vi "Read User Devices.vi"(8 "error in (no error)":errorcluster, 11 "Platforms":refnum<class "PlatformManager.lvclass">) -> (0 "error out":errorcluster, 3 "User Devices":refnum<class "Device.lvclass">[](array[class]))   [LabVIEW 2020, in "PicoG-App.lvlib" / "picoG.lvclass"]
uses:
  picoG.lvclass
  Device/Device.lvclass
  Builds/picoG/ppl/PicoG-Core.lvlibp/PicoG-Processor/PicoG-Core/PlatformManager/PlatformManager.lvclass
  <vilib>/Utility/config.llb/Read Key (I32).vi
  PicoG-App.lvlib
  <vilib>/Utility/config.llb/NI_LVConfig.lvlib
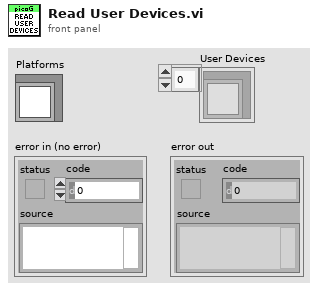
[diagram p1: front panel]
types:
  T1 = typedef "PicoG-App.lvlib/Paths.ctl" = cluster{"User picoG":path, "System picoG":path, "User Config":path, "System Config":path}
  T2 = typedef "NI_LVConfig.lvlib/Config Data RefNum.ctl" = refnum<k1>
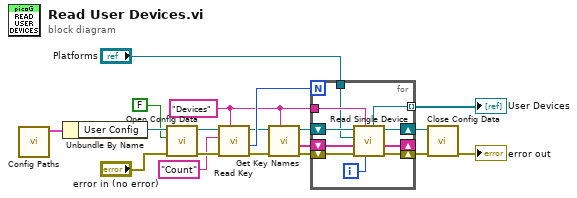
[diagram p0: block diagram]
diagram:
  w2 = "Devices" ("key")
  n1 = call "Config Paths.vi"() -> ("Paths"=w19:T1)  [unwired: 8 in, 3 out]
  n2 = Unbundle By Name(w19) -> ("User Config"=w18:path)
  n3 = call <vilib>:"Open Config Data.vi"("error in (no error)"="error in (no error)", "create file if necessary (T)"=FALSE, "configuration file path"=w18) -> ("error out"=w15:errorcluster, "refnum"=w16:T2)  [unwired: 6 in, 1 out]
  n4 = call-poly <vilib>:"Read Key.vi"("section"=w2, "error in (no error)"=w15, "key"="Count", "refnum"=w16) -> ("error out"=w6:errorcluster, "value"=w13:i32, "refnum out"=w7:T2)  [unwired: 4 in, 1 out]
  n5 = call <vilib>:"Get Key Names.vi"("section"=w2, "error in (no error)"=w6, "refnum"=w7) -> ("error out"=w4:errorcluster, "key names"=w5:string[], "refnum out"=w3:T2)  [unwired: 5 in, 1 out]
  n6 = for {
    N: w13 -> [_]
    shift-right: [w26] -> w10
    shift-left: w4 -> [w28]
    shift-right: [w25] -> w11
    shift-left: w3 -> [w29]
    tunnel: w2 -> [w24]
    tunnel: [w22] -> w12 mode=indexing
    shift-right: [w21] -> _
    shift-left: w5 -> [w23]
    tunnel: "Platforms" -> [w20]
    i -> [w27]
    n7 = call "Read Single Device.vi"("Index"=w27, "Section"=w24, "error in (no error)"=w28, "Key Names"=w23, "Platforms"=w20, "refnum"=w29) -> ("error out"=w26:errorcluster, "Remaining Key Names"=w21:string[], "refnum out"=w25:T2, "Device"=w22:refnum<class "Device.lvclass">)  [unwired: 2 in]
  }
  "User Devices" <- w12
  n8 = call <vilib>:"Close Config Data.vi"("error in (no error)"=w10, "refnum"=w11) -> ("error out"=→"error out":errorcluster)  [unwired: 8 in, 1 out]
